vi "GE 5565PIORC.DMA.Poll for Done Signal.vi"(8 "error in (no error)":errorcluster, 10 "timeout ms (1000)":u32=1000, 11 "GE 5565PIORC in":refnum<class "GE 5565PIORC.lvclass">) -> (0 "error out":errorcluster, 2 "timed out?":bool, 3 "GE 5565PIORC out":refnum<class "GE 5565PIORC.lvclass">)   [LabVIEW 2024, in "GE 5565PIORC.lvclass"]
doc: "Polls the DMA Inactive register until the DMA transfer is complete, or the specified <b>timeout ms</b> has been reached."
uses:
  GE 5565PIORC.lvclass
  GE 5565PIORC.lvclass/GE 5565PIORC.ctl
  Properties/Registers/GE 5565PIORC.Registers.DMACSR0.Channel 0 Inactive.Get.vi
  Properties/Registers/GE 5565PIORC.Registers.Local Configuration.Read.vi
  Properties/Registers/GE 5565PIORC.Registers.Local Configuration.Read (U8).vi
  GE 5565PIORC.Bit Manipulation.Get Bit.vi
  GE 5565PIORC.Bit Manipulation.Get Bit (U8).vi
  GE 5565PIORC.Registers.Read.vi
  GE 5565PIORC.Registers.Read (U8).vi
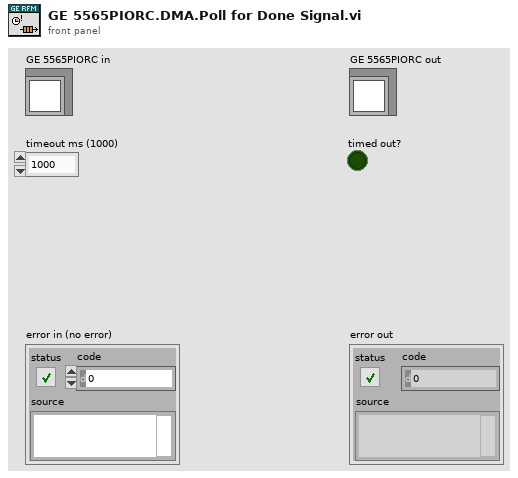
[diagram p1: front panel]
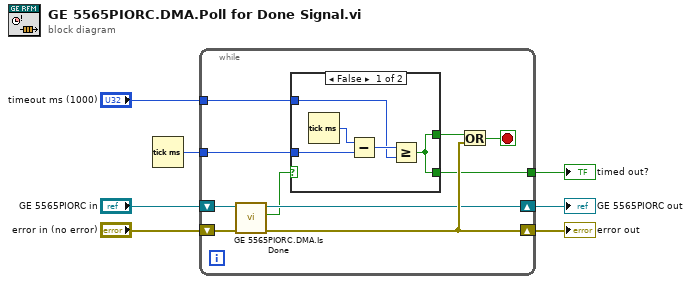
[diagram p0: block diagram]
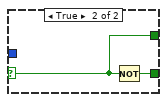
[diagram p2: hidden frame]
diagram:
  n1 = Tick Count (ms)() -> (millisecond timer value=w3:u32)
  n2 = while {
    shift-right: [w10] -> w6
    shift-left: "GE 5565PIORC in" -> [w13]
    shift-right: [w11] -> w4
    shift-left: "error in (no error)" -> [w12]
    tunnel: "timeout ms (1000)" -> [w16]
    tunnel: w3 -> [w17]
    tunnel: [w8] -> w1
    stop <- w14 stop-if-true
    n3 = call "GE 5565PIORC.DMA.Is Done.vi"("error in (no error)"=w12, "GE 5565PIORC in"=w13) -> ("error out"=w11:errorcluster, "dma done?"=w9:bool, "GE 5565PIORC out"=w10:refnum<class "GE 5565PIORC.lvclass">)  [unwired: 7 in]
    n4 = case shown="False" w9 {
      selector: w9 -> [_ w23]
      tunnel: w17 -> [w21 _]
      tunnel: w16 -> [w19 _]
      tunnel: [w18 w24] -> w8
      tunnel: [w18 w23] -> w15
      frame False {
        n5 = Tick Count (ms)() -> (millisecond timer value=w22:u32)
        n6 = Subtract(x=w22, y=w21) -> (x-y=w20:u32)
        n7 = Greater Or Equal?(x=w20, y=w19) -> (x >= y?=w18:bool)
      }
      frame True {
        n8 = Not(x=w23) -> (.not. x?=w24:bool)
      }
    }
    n9 = Or(x=w15, y=w11) -> (x .or. y?=w14:bool)
  }
  "GE 5565PIORC out" <- w6
  "error out" <- w4
  "timed out?" <- w1
